vi "ActorNR.vi"(10 "Startup Message":refnum<class "MSG.lvclass">, 11 "Controller":refnum<class "Controller.lvclass">) -> ()   [LabVIEW 2016, in "Controller.lvclass"]
doc: "A Non-Reentrant version of Actor.vi. One can switch between the two by renaming (Actor.vi <-> ActorNR.vi) and changing the reentrancy setting (Shared-Reentrant <-> Non-Reentrant)."
uses:
  Controller.lvclass
  <vilib>/drjdpowell/Messenging/Core Messages/Message/MSG.lvclass
  <vilib>/drjdpowell/Messenging/Parallel Process/Actor type 2/Actor type2.lvclass
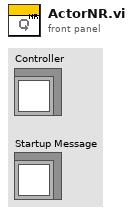
[diagram p1: front panel]
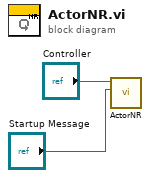
[diagram p0: block diagram]
diagram:
  n1 = call-parent "ActorNR.vi"("Startup Message"="Startup Message", "Actor type2"="Controller") -> ()  [unwired: 10 in]
